vi "IT8800-Configure Operation Value.vi"(8 "error in":errorcluster, 9 "Values (0)":dbl format="%#.3g", 10 "Value Type (0:Current)":T2, 11 "IT8800 Setting In In":T1={"VISA Resource Name"="", "Baud Rate"=19200, "Stop Bits"=20, "Wait For Read(ms)"=0, "Interface Type"=enum."VXI", "Limits"=[]} {"Stop Bits" items=["1.0"=10, "2.0"=20]; "Baud Rate" items=["2400"=2400, "4800"=4800, "9600"=9600, "19200"=19200]}) -> (0 "error out":errorcluster, 3 "IT8800 Setting In Out":T1={"VISA Resource Name"="", "Baud Rate"=19200, "Stop Bits"=20, "Wait For Read(ms)"=0, "Interface Type"=enum."VXI", "Limits"=[]} {"Stop Bits" items=["1.0"=10, "2.0"=20]; "Baud Rate" items=["2400"=2400, "4800"=4800, "9600"=9600, "19200"=19200]})   [LabVIEW 2018]
doc: "Configures the current, voltage, power or conductance depending the instrument operation mode.\n\n<b>Note:</b>\nIn these modes, only the following values are allowed.\n1) CC -Current\n2) CV -Voltage\n3) CP -Power\n4) CR- Conductance\n5) CC+CV -Current & Voltage\n6) CR+CV -Conductance & Voltage"
uses:
  Data Def/IT8800-Operation Mode.ctl
  Data Def/IT8800-Setting.ctl
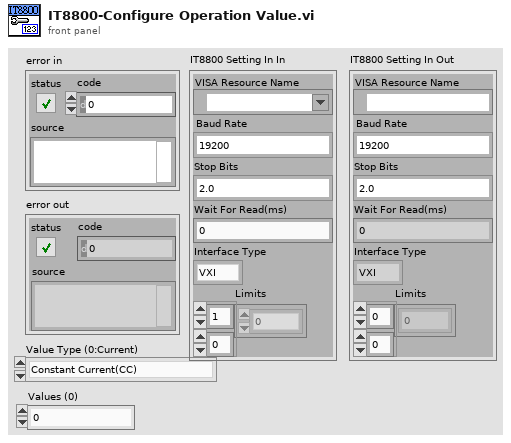
[diagram p1: front panel]
types:
  T1 = typedef "IT8800-Setting.ctl" = cluster{"VISA Resource Name":refnum<visa-resource-name>, "Baud Rate":u32, "Stop Bits":u16, "Wait For Read(ms)":u32, "Interface Type":enum16{"Unknow", "GPIB", "VXI", "GPIB-VXI", "Serial", "PXI", "TCPIP", "USB", "FireWire"}, "Limits":dbl[][]}
  T2 = typedef "IT8800-Operation Mode.ctl" = enum16{"Constant Current(CC)", "Constant Voltage(CV)", "Constant Power(CP)", "Constant Resistance(CR)"}
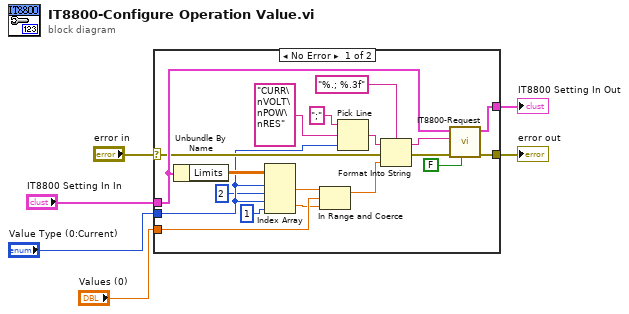
[diagram p0: block diagram]
diagram:
  n1 = case shown="No Error" "error in" {
    selector: "error in" -> [w10 w27]
    tunnel: [w19 w27] -> w6
    tunnel: [w18 w26] -> w5
    tunnel: "IT8800 Setting In In" -> [w16 w26]
    tunnel: "Values (0)" -> [w15 _]
    tunnel: "Value Type (0:Current)" -> [w9 _]
    frame No Error {
      n2 = Unbundle By Name(w16) -> ("Limits"=w11:dbl[][])
      n3 = Index Array(array=w11, index (row) #1=w9, index (col) #1=2 ("index (row)"), index (row) #2=w9, index (col) #2=1 ("disabled index (row)")) -> (element #1=w13:dbl, element #2=w12:dbl)
      n4 = In Range and Coerce(upper limit=w13, x=w15, lower limit=w12) -> (coerced(x)=w14:dbl)  [unwired: 1 out]
      n5 = Pick Line(string ("")=";", multi-line string="CURR\nVOLT\nPOW\nRES", line index=w9) -> (output string=w23:string)
      n6 = Format Into String(format string="%.; %.3f", initial string=w23, error in=w10, w14) -> (resulting string=w20:string, error out=w21:errorcluster)
      n7 = call "IT8800-Request.vi"("Response?"=FALSE, "error in"=w21, "Command"=w20, "IT8800 Setting In In"=w16) -> ("error out"=w19:errorcluster, "IT8800 Setting In Out"=w18:T1)  [unwired: 5 in, 1 out]
    }
    frame Error {
    }
  }
  "error out" <- w6
  "IT8800 Setting In Out" <- w5
